vi "Read angles.lvclass.vi"(8 "error in (no error)":errorcluster, 11 "AG in":refnum<class "AG.lvclass">) -> (0 "error out":errorcluster, 2 "angles.lvclass":refnum<class "angles.lvclass">, 3 "AG out":refnum<class "AG.lvclass">)   [LabVIEW 2018, in "AG.lvclass"]
uses:
  AG.lvclass
  Device/angles/angles.lvclass
  AG.lvclass/AG.ctl
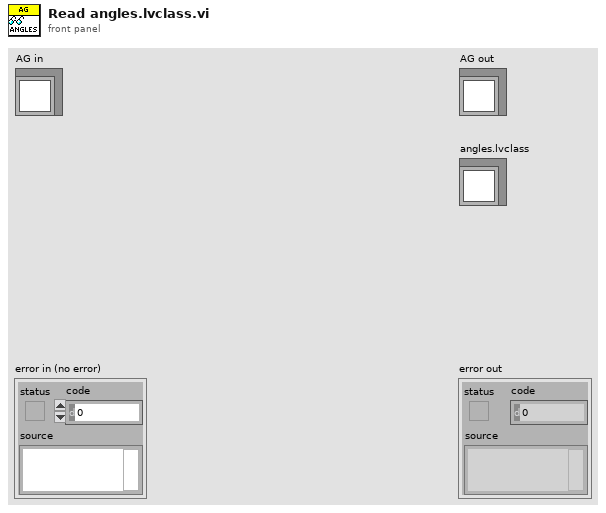
[diagram p1: front panel]
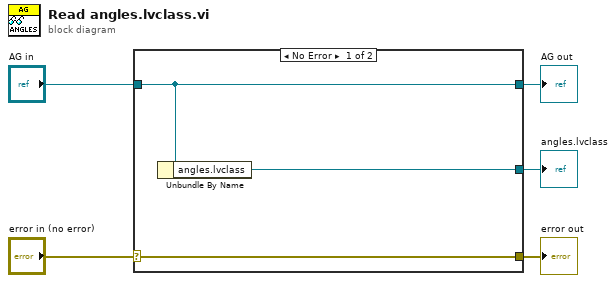
[diagram p0: block diagram]
diagram:
  n1 = case shown="No Error" "error in (no error)" {
    selector: "error in (no error)" -> [w8 w9]
    tunnel: [w8 w9] -> w4
    tunnel: [w7 w10] -> w2
    tunnel: "AG in" -> [w7 w10]
    tunnel: [w6 _] -> w1
    frame No Error {
      n2 = Unbundle By Name(w7) -> ("angles.lvclass"=w6:refnum<class "angles.lvclass">)
    }
    frame Error {
    }
  }
  "error out" <- w4
  "AG out" <- w2
  "angles.lvclass" <- w1
